vi "DeviceLostCallback.vi"(4 "User Parameter":variant, 6 "Control Ref":refnum<k7>, 7 "Event Common Data":T1) -> ()   [LabVIEW 2010]
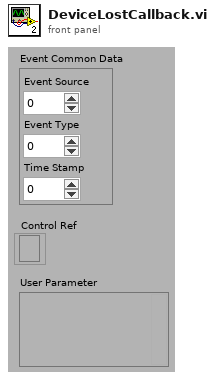
[diagram p1: front panel]
types:
  T1 = cluster{"Event Source":i32, "Event Type":u32, "Time Stamp":u32}
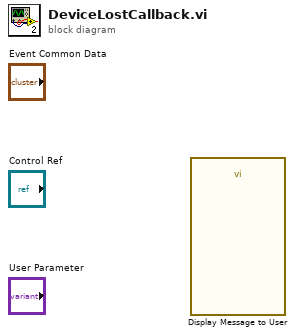
[diagram p0: block diagram]
diagram:
  n1 = call "Display Message to User"() -> ()  [unwired: 10 in, 2 out]
